vi "PH_Cont-601k_PSU.panel.vi"(0 "object ref":refnum<vi>, 5 "error in (no error)":errorcluster) -> (19 "error out":errorcluster)   [LabVIEW 2014, in "PH_Cont-601k_PSU.lvlib"]
doc: "This a GUI.\n\nLicense Agreement for this software:\n\nCopyright (C)\nGesellschaft für Schwerionenforschung, GSI\nPlanckstr. 1\n64291 Darmstadt\nGermany\n\nContact: D.Beck@gsi.de \n\nThis program is free software; you can redistribute it and/or modify it under the terms of the GNU General Public License as published by the Free Software Foundation; either version 2 of the license, or (at your option) any later version.\n\nThis program is distributed in the hope that it will be useful, but WITHOUT ANYW ARRANTY; without even the implied warranty of MERCHANTABILITY or FITNESS FOR A PARTICULAR PURPOSE. See the GNU General License for more details (http://www.gnu.org).\n\nGesellschaft für Schwerionenforschung, GSI\nPlanckstr. 1, 64291 Darmstadt, Germany\nFor all questions and ideas contact: M.Richter@gsi.de, H.Brand@gsi.de or D.Beck@gsi.de.\nLast update: 18-DEC-2002"
uses:
  PH_Cont-601k_PSU.lvlib
  PH_Cont-601k_PSU.Mode.ctl
  PH_Cont-601k_PSU.Configuration.ctl
  PH_Cont-601k_PSU.Device Status.ctl
  PH_Cont-601k_PSU.Device Informaton.ctl
  PH_Cont-601k_PSU.Readyness.ctl
  PH_Cont-601k_PSU.Readyness Program.ctl
  PH_Cont-601k_PSU.Readyness Device.ctl
  PH_Cont-601k_PSU.GUI Refs.ctl
  CSCore/CSObj/CSObj.lvlib
  PH_Common/PH_Common.lvlib
  CSCore/CSSystem/CSSystemLib/CSSystemLib.lvlib
  PH_Class/PH_Class.lvlib
panel:
  in  "Tab Control":T1(tab)
  out "PSU On":u32(colorbox)=16860
  out "Interlock Indicator":u32(colorbox)=16860
  in  "Interlock":bool
  in  "Charge":bool
  in  "Mode":T2
  in  "Configuration":T3 items=["Ch intl, Fl intl, QSw intl", "Ch intl, Fl intl, QSw ext", "Ch intl, Fl ext, QSw intl", "Ch intl, Fl ext, QSw ext", "Ch ext, Fl int, QSw int", "Ch ext, Fl int, QSw ext", "Ch ext, Fl ext, QSw int", "Ch ext, Fl ext, QSw ext"]
  in  "Voltage [V]":u16 max=2000 step=10
  in  "Flash Interval [s]":dbl min=5.0 max=60.0 step=1.0
  out "Device Status":T4={"State"=0, "Interlocks"=[], "EOC"=16860, "Flashlamp Counter"=0, "error message"=""} {"State" items=["STOP: Stop Mode"=0, "STOP: Retrieve laser head serial number"=2, "STOP: Read flash and Q-switch counters"=3, "STOP: Keyswitch off"=5, "STOP: Delay for SmartBoard to get ready"=4, "STOP: SmartBoard download initialization"=6, "STOP: Retrieve SmartBoard version information"=7, "STOP: Retrieve all infos from SmartBoard"=8, "STOP: Stop Initialization"=10, "STOP: At Power-ON, found RUN, waiting for STOP"=15, "STOP: Idle, waiting for commands"=20, "STOP: Init laser head downloading process"=25, "STOP: Retrieve SmartBoard EEPROM location"=27, "STOP: Download laser head data"=30, "STOP: Initialize Power On Self Tests"=35, "STOP: Power On Self Test: Wait for pump to turn on"=40, "STOP: Power On Self Test: Wait for shutter to close"=45, "STOP: Power On Self Test: Wait for shutter to open"=50, "STANDBY: Standby Mode"=100, "STANDBY: Standby Initialization"=110, "STANDBY: Waiting for SmartBoard to complete a task"=113, "STANDBY: Idle, waiting for commands"=120, "STANDBY: Waiting for Smart Board to complete a task"=123, "STANDBY: At Power-ON, found READY. Waiting for STANDBY"=130, "READY: Ready Mode"=200, "READY: Ready Mode Initialization"=205, "READY: Begin Charging"=206, "READY: Wait for initial capacitor charge"=207, "READY: Charging"=208, "READY: Initial charge completion"=209, "READY: Idle, waiting for commands"=210, "READY: Uploading of paramters to the laser head"=215, "EMISSION: Emission Mode"=300, "EMISSION: Idle, waiting for commands"=310, "EMISSION: Waiting for shutter to close"=311, "EMISSION: Waiting to set pyro"=313, "EMISSION: Servo control to hold value"=315, "EMISSION: Servo context monitoring"=320, "EMISSION: Initialization for laser head pyro gein adjustment"=330, "EMISSION: Pyro gain adjustment - step 1"=335, "EMISSION: Pyro gain adjustment - step 2"=340, "EMISSION: Pyro gain adjustment - step 3"=345, "EMISSION: Pyro gain adjustment complete"=350, "ERROR: Error Mode"=400, "ERROR: Initialization for error mode"=405, "ERROR: Cooling Error - wating for STOP"=410, "ERROR: Error control for laser head not initialized fault."=415, "ERROR: Error control for TS-485 (Smart Bus) fault."=420, "ERROR: Error control for cover interlocks"=425, "ERROR: Watchdog Timeout"=435]}
  out "Power On":u32(colorbox)=16860
  in  "Reset Error":bool
  in  "Expert working":bool
  out "Device Error":errorcluster caption="Error"
  out "Hard- and Software":T5={"VISA resource"="COM1", "Driver Revision"="", "Firmware Revision"=""}
  out "Readyness":T6
  in  "Delete":bool
  in  "Exit":bool
  # "PCS"
  # "3.40"
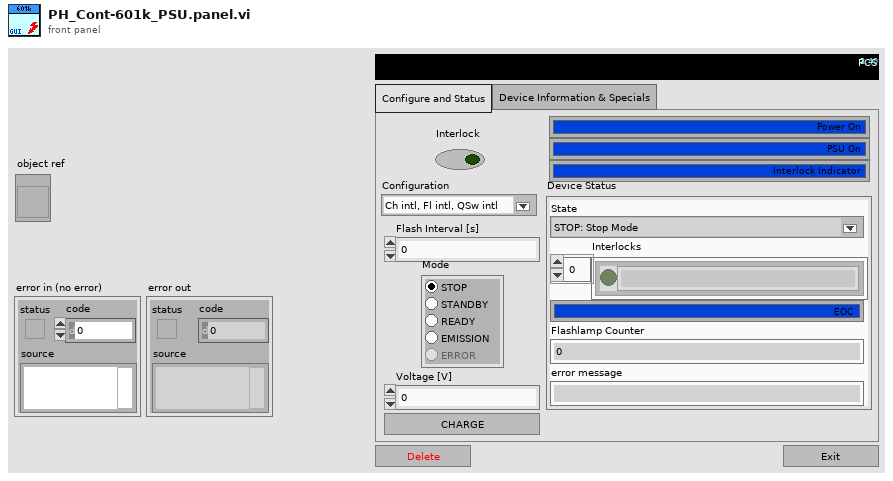
[diagram p1: front panel]
types:
  T1 = enum32{"Configure and Status", "Device Information & Specials"}
  T2 = typedef "PH_Cont-601k_PSU.lvlib/PH_Cont-601k_PSU.Mode.ctl" = enum32{"STOP", "STANDBY", "READY", "EMISSION", "ERROR"}
  T3 = typedef "PH_Cont-601k_PSU.lvlib/PH_Cont-601k_PSU.Configuration.ctl" = u16
  T4 = typedef "PH_Cont-601k_PSU.lvlib/PH_Cont-601k_PSU.Device Status.ctl" = cluster{"State":u16, "Interlocks":cluster{"on/off":bool, "Explanation":string}[], "EOC":u32, "Flashlamp Counter":u32, "error message":string}
  T5 = typedef "PH_Cont-601k_PSU.lvlib/PH_Cont-601k_PSU.Device Informaton.ctl" = cluster{"VISA resource":refnum<visa-resource-name>, "Driver Revision":string, "Firmware Revision":string}
  T6 = typedef "PH_Cont-601k_PSU.lvlib/PH_Cont-601k_PSU.Readyness.ctl" = cluster{"Program":T7, "Device":T8}
  T7 = typedef "PH_Cont-601k_PSU.lvlib/PH_Cont-601k_PSU.Readyness Program.ctl" = enum32{"OFF", "POWER", "INTERLOCK"}
  T8 = typedef "PH_Cont-601k_PSU.lvlib/PH_Cont-601k_PSU.Readyness Device.ctl" = enum32{"OFF", "CONNECTING", "CONNECTED", "OPERATING", "EOC", "ERROR"}
  T9 = typedef "PH_Cont-601k_PSU.lvlib/PH_Cont-601k_PSU.GUI Refs.ctl" = cluster{"Power On":refnum<vi>, "Hard- and Software":refnum<vi>, "Device Status":refnum<vi>, "Device Error":refnum<vi>, "Configuration":refnum<vi>, "Flash Interval [s]":refnum<vi>, "Interlock":refnum<vi>, "Interlock Indicator":refnum<vi>, "Voltage [V]":refnum<vi>, "Readyness":refnum<vi>, "Mode":refnum<vi>, "Reset Error":refnum<vi>, "Expert working":refnum<vi>, "Charge":refnum<vi>, "PSU On":refnum<vi>}
  T10 = typedef "PH_Cont-601k_PSU.lvlib/PH_Cont-601k_PSU.i attribute.ctl" = cluster{"GUI Refs":T9, "Interlock":bool, "Service ID applied Voltage":i32, "Device Settings":cluster{"Configuration":T3, "Flash Interval [s]":dbl, "Mode":T2, "Voltage [V]":u16, "Charge":bool, "VISA resource name":refnum<visa-resource-name>}, "Readyness":T6, "Information":cluster{"VISA resource name":refnum<visa-resource-name>, "Tagname Power On":string, "Interlock":cluster{"Instance":string, "Tagname":string}, "Limits [V]":cluster{"Lower":dbl, "Upper":dbl}, "Tagname PSU On":string}, "R2S":bool, "Charge is allowed":bool}
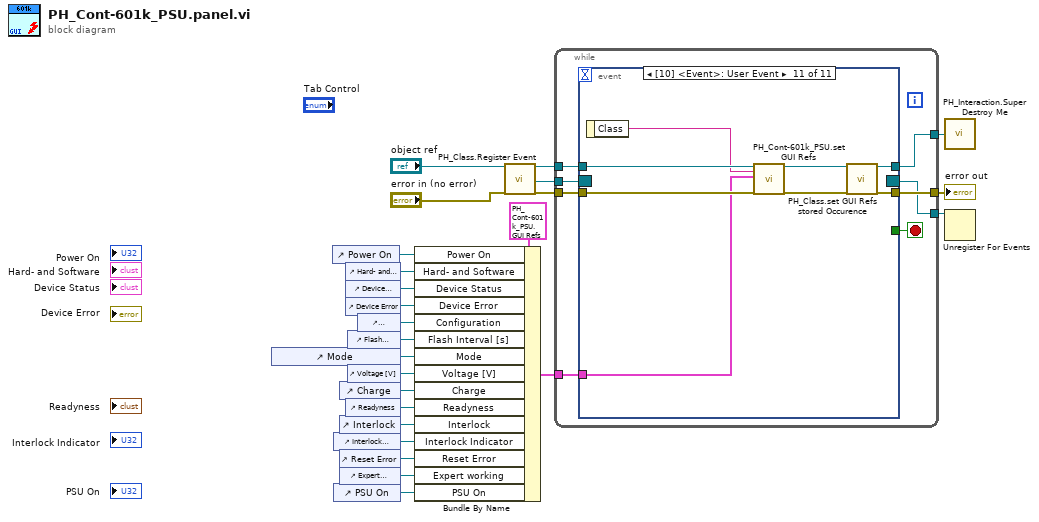
[diagram p0: block diagram]
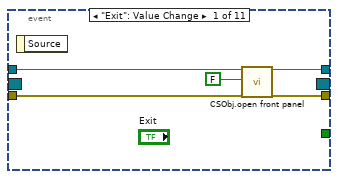
[diagram p2: hidden frame]
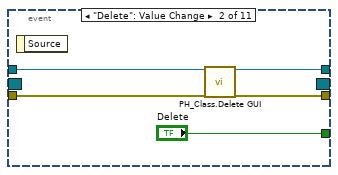
[diagram p3: hidden frame]
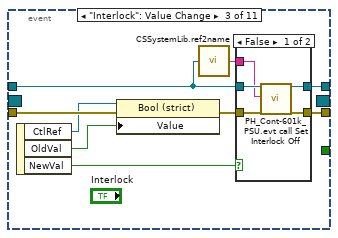
[diagram p4: hidden frame]
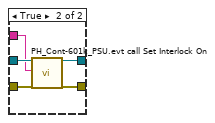
[diagram p5: hidden frame]
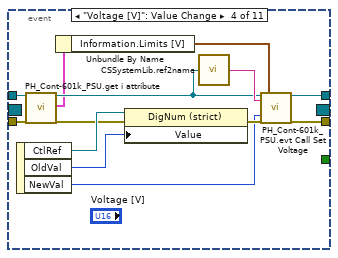
[diagram p6: hidden frame]
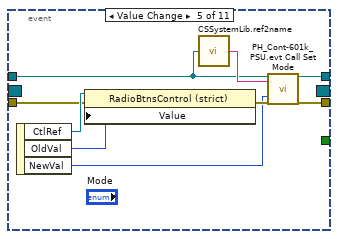
[diagram p7: hidden frame]
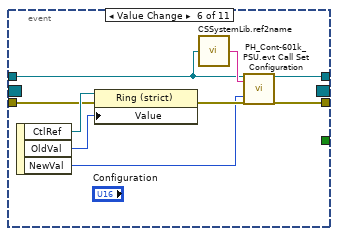
[diagram p8: hidden frame]
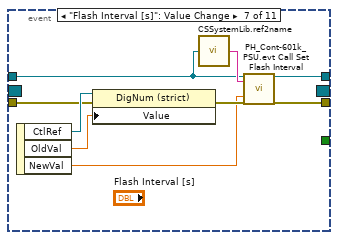
[diagram p9: hidden frame]
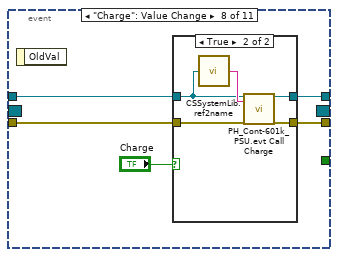
[diagram p10: hidden frame]
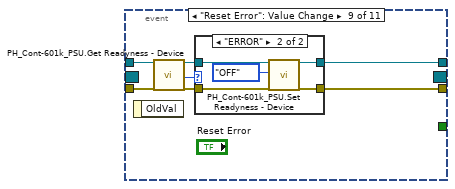
[diagram p12: hidden frame]
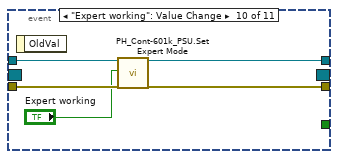
[diagram p14: hidden frame]
diagram:
  n1 = control-ref of="Mode"() -> (w21:refnum<vi>)
  n2 = control-ref of="Power On"() -> (w23:refnum<vi>)
  n3 = control-ref of="Interlock Indicator"() -> (w16:refnum<vi>)
  n4 = control-ref of="PSU On"() -> (w1:refnum<vi>)
  n5 = control-ref of="Charge"() -> (w10:refnum<vi>)
  n6 = control-ref of="Interlock"() -> (w17:refnum<vi>)
  n7 = control-ref of="Reset Error"() -> (w11:refnum<vi>)
  n8 = control-ref of="Expert working"() -> (w12:refnum<vi>)
  n9 = control-ref of="Hard- and Software"() -> (w18:refnum<vi>)
  n10 = control-ref of="Device Status"() -> (w13:refnum<vi>)
  n11 = control-ref of="Device Error"() -> (w22:refnum<vi>)
  n12 = control-ref of="Readyness"() -> (w14:refnum<vi>)
  n13 = control-ref of="Flash Interval [s]"() -> (w19:refnum<vi>)
  n14 = control-ref of="Voltage [V]"() -> (w15:refnum<vi>)
  n15 = control-ref of="Configuration"() -> (w20:refnum<vi>)
  n16 = Bundle By Name(cluster=T9 {"Power On"=refnum, "Hard- and Software"=refnum, "Device Status"=refnum, "Device Error"=refnum, "Configuration"=refnum, "Flash Interval [s]"=refnum, "Interlock"=refnum, "Interlock Indicator"=refnum, "Voltage [V]"=refnum, "Readyness"=refnum, "Mode"=refnum, "Reset Error"=refnum, "Expert working"=refnum, "Charge"=refnum, "PSU On"=refnum} ("GUI Refs"), "Power On"=w23, "Hard- and Software"=w18, "Device Status"=w13, "Device Error"=w22, "Configuration"=w20, "Flash Interval [s]"=w19, "Mode"=w21, "Voltage [V]"=w15, "Charge"=w10, "Readyness"=w14, "Interlock"=w17, "Interlock Indicator"=w16, "Reset Error"=w11, "Expert working"=w12, "PSU On"=w1) -> (w2:T9)
  n17 = call "PH_Class.Register Event.vi"("i ref in"="object ref", "error in (no error)"="error in (no error)") -> ("i ref out"=w8:refnum<vi>, "Event Registration Refnum"=w6:refnum<event-registration>, "error out"=w7:errorcluster)  [unwired: 15 in]
  n18 = while {
    tunnel: w8 -> [w30]
    tunnel: [w29] -> w25
    tunnel: w7 -> [w32]
    tunnel: [w31] -> w24
    tunnel: w6 -> [w28]
    tunnel: [w27] -> w5
    tunnel: w2 -> [w26]
    stop <- w33 stop-if-true
    n19 = event shown="[10] <Event>: User Event" {
      selector: w28 -> [_ _ _ _ _ _ _ _ _ _ _]
      dyn-events: [_ _ _ _ _ _ _ _ _ _ _] -> w27
      timeout: _ -> [_ _ _ _ _ _ _ _ _ _ _]
      tunnel: [_ "Delete" _ _ _ _ _ _ _ _ _] -> w33
      tunnel: w30 -> [w35 w40 w49 w66 w77 w87 w95 w105 w119 w133 w141]
      tunnel: w32 -> [w38 w39 w46 w71 w76 w86 w94 w104 w118 w132 w140]
      tunnel: [w37 w42 w51 w74 w83 w92 w101 w106 w120 w130 w137] -> w31
      tunnel: [w34 w41 w52 w75 w84 w93 w102 w107 w121 w131 w136] -> w29
      tunnel: w26 -> [_ _ _ _ _ _ _ _ _ _ w135]
      event "Exit": Value Change {
        n20 = event-data() -> ()  [unwired: 1 in, 1 out]
        n21 = call "CSObj.open front panel.vi"("i ref in"=w35, "frontPanelOpen"=FALSE ("front panel open"), "error in (no error)"=w38) -> ("i ref out"=w34:refnum<vi>, "error out"=w37:errorcluster)  [unwired: 15 in]
      }
      event "Delete": Value Change {
        n22 = event-data() -> ()  [unwired: 1 in, 1 out]
        n23 = call "PH_Class.Delete GUI.vi"("VI in"=w40, "error in (no error)"=w39) -> ("VI out"=w41:refnum<vi>, "error out"=w42:errorcluster)  [unwired: 16 in]
      }
      event "Interlock": Value Change {
        n24 = event-data() -> ("CtlRef"=w45:refnum<vi>, "OldVal"=w44:bool, "NewVal"=w50:bool)  [unwired: 1 in]
        n25 = property class="Bool (strict)"(reference=w45, error in=w46, "Value"=w44) -> (error out=w47:errorcluster)  [unwired: 1 out]
        n26 = call "CSSystemLib.ref2name.vi"("obj refnum"=w49) -> ("name"=w48:string)
        n27 = case shown="False" w50 {
          tunnel: w49 -> [w57 w62]
          tunnel: w47 -> [w56 w61]
          tunnel: [w55 w60] -> w52
          tunnel: [w54 w59] -> w51
          tunnel: w48 -> [w53 w58]
          frame False {
            n28 = call "PH_Cont-601k_PSU.evt call Set Interlock Off.vi"("i ref in"=w57, "Instance name"=w53, "error in"=w56) -> ("i ref out"=w55:refnum<vi>, "error out"=w54:errorcluster)  [unwired: 15 in]
          }
          frame True {
            n29 = call "PH_Cont-601k_PSU.evt call Set Interlock On.vi"("i ref in"=w62, "Instance name"=w58, "error in"=w61) -> ("i ref out"=w60:refnum<vi>, "error out"=w59:errorcluster)  [unwired: 15 in]
          }
        }
      }
      event "Voltage [V]": Value Change {
        n30 = event-data() -> ("CtlRef"=w70:refnum<vi>, "OldVal"=w69:u16, "NewVal"=w68:u16)  [unwired: 1 in]
        n31 = call "PH_Cont-601k_PSU.get i attribute.vi"("i ref in"=w66, "error in (no error)"=w71) -> ("i ref out"=w65:refnum<vi>, "i attribute"=w64:T10, "error out"=w67:errorcluster)  [unwired: 15 in]
        n32 = Unbundle By Name(w64) -> ("Information.Limits [V]"=w63:cluster{"Lower":dbl, "Upper":dbl})
        n33 = property class="DigNum (strict)"(reference=w70, error in=w67, "Value"=w69) -> (error out=w72:errorcluster)  [unwired: 1 out]
        n34 = call "CSSystemLib.ref2name.vi"("obj refnum"=w65) -> ("name"=w73:string)
        n35 = call "PH_Cont-601k_PSU.evt Call Set Voltage.vi"("i ref in"=w65, "Instance name"=w73, "Voltage to set [V]"=w68, "error in"=w72, "Limits [V]"=w63) -> ("i ref out"=w75:refnum<vi>, "error out"=w74:errorcluster)  [unwired: 13 in]
      }
      event Value Change {
        n36 = event-data() -> ("CtlRef"=w80:refnum<vi>, "OldVal"=w79:T2, "NewVal"=w78:T2)  [unwired: 1 in]
        n37 = property class="RadioBtnsControl (strict)"(reference=w80, error in=w76, "Value"=w79) -> (error out=w81:errorcluster)  [unwired: 1 out]
        n38 = call "CSSystemLib.ref2name.vi"("obj refnum"=w77) -> ("name"=w82:string)
        n39 = call "PH_Cont-601k_PSU.evt Call Set Mode.vi"("i ref in"=w77, "Instance name"=w82, "Mode to set"=w78, "error in"=w81) -> ("i ref out"=w84:refnum<vi>, "error out"=w83:errorcluster)  [unwired: 14 in]
      }
      event Value Change {
        n40 = event-data() -> ("CtlRef"=w89:refnum<vi>, "OldVal"=w88:T3, "NewVal"=w85:T3)  [unwired: 1 in]
        n41 = property class="Ring (strict)"(reference=w89, error in=w86, "Value"=w88) -> (error out=w90:errorcluster)  [unwired: 1 out]
        n42 = call "CSSystemLib.ref2name.vi"("obj refnum"=w87) -> ("name"=w91:string)
        n43 = call "PH_Cont-601k_PSU.evt Call Set Configuration.vi"("i ref in"=w87, "Instance name"=w91, "Configuration to set"=w85, "error in"=w90) -> ("i ref out"=w93:refnum<vi>, "error out"=w92:errorcluster)  [unwired: 14 in]
      }
      event "Flash Interval [s]": Value Change {
        n44 = event-data() -> ("CtlRef"=w98:refnum<vi>, "OldVal"=w97:dbl, "NewVal"=w96:dbl)  [unwired: 1 in]
        n45 = property class="DigNum (strict)"(reference=w98, error in=w94, "Value"=w97) -> (error out=w99:errorcluster)  [unwired: 1 out]
        n46 = call "CSSystemLib.ref2name.vi"("obj refnum"=w95) -> ("name"=w100:string)
        n47 = call "PH_Cont-601k_PSU.evt Call Set Flash Interval.vi"("i ref in"=w95, "Instance name"=w100, "Flash Interval [s]"=w96, "error in"=w99) -> ("i ref out"=w102:refnum<vi>, "error out"=w101:errorcluster)  [unwired: 14 in]
      }
      event "Charge": Value Change {
        n48 = event-data() -> ()  [unwired: 1 in, 1 out]
        n49 = case shown="True" "Charge" {
          tunnel: [w109 w114] -> w107
          tunnel: [w108 w113] -> w106
          tunnel: w105 -> [w109 w111]
          tunnel: w104 -> [w108 w110]
          frame False {
          }
          frame True {
            n50 = call "CSSystemLib.ref2name.vi"("obj refnum"=w111) -> ("name"=w112:string)
            n51 = call "PH_Cont-601k_PSU.evt Call Charge.vi"("i ref in"=w111, "Instance name"=w112, "error in"=w110) -> ("i ref out"=w114:refnum<vi>, "error out"=w113:errorcluster)  [unwired: 15 in]
          }
        }
      }
      event "Reset Error": Value Change {
        n52 = event-data() -> ()  [unwired: 1 in, 1 out]
        n53 = call "PH_Cont-601k_PSU.Get Readyness - Device.vi"("VI in"=w119, "error in (no error)"=w118) -> ("VI out"=w117:refnum<vi>, "Readyness - Device"=w115:T8, "error out"=w116:errorcluster)  [unwired: 15 in]
        n54 = case shown="\"ERROR\"" w115 {
          tunnel: [w123 w128] -> w121
          tunnel: [w122 w127] -> w120
          tunnel: w117 -> [w123 w126]
          tunnel: w116 -> [w122 w125]
          frame Default {
          }
          frame "ERROR" {
            n55 = call "PH_Cont-601k_PSU.Set Readyness - Device.vi"("VI in"=w126, "Readyness - Device"=PH_Cont-601k_PSU.Readyness_Device."OFF", "error in (no error)"=w125) -> ("VI out"=w128:refnum<vi>, "error out"=w127:errorcluster)  [unwired: 15 in]
          }
        }
      }
      event "Expert working": Value Change {
        n56 = event-data() -> ()  [unwired: 1 in, 1 out]
        n57 = call "PH_Cont-601k_PSU.Set Expert Mode.vi"("VI in"=w133, "Expert working"="Expert working", "error in (no error)"=w132) -> ("VI out"=w131:refnum<vi>, "error out"=w130:errorcluster)  [unwired: 15 in]
      }
      event User Event {
        n58 = event-data() -> ("Class"=w134:string)  [unwired: 1 in]
        n59 = call "PH_Cont-601k_PSU.set GUI Refs.vi"("VI in"=w141, "Class"=w134, "GUI Refs"=w135, "error in (no error)"=w140) -> ("VI out"=w139:refnum<vi>, "error out"=w138:errorcluster)  [unwired: 14 in]
        n60 = call "PH_Class.set GUI Refs stored Occurence.vi"("i ref in"=w139, "error in (no error)"=w138) -> ("i ref out"=w136:refnum<vi>, "error out"=w137:errorcluster)  [unwired: 16 in]
      }
    }
  }
  "error out" <- w24
  n61 = call "PH_Interaction.Super Destroy Me.vi"("i ref out"=w25) -> ()
  n62 = Unregister For Events(event registration refnum=w5) -> ()  [unwired: 1 in, 1 out]
